vi "Iconos Indicador actual Test.vi"(8 "Test":T1 items=["Power", "Oscilloscope", "Pulse Generator", "Link FT232", "Default Reg", "W/R REG", "ADC", "Max P Min N", "Min P Max N", "Digital Offset", "Analog Offset", "Rate Scan", "Rate Scan ADD"], 9 "Icon":T2, 10 "Vasic Actual":i32, 11 "Result Test IN":T3 {"Voltage ASIC" format="%1_3g"}) -> (3 "Result Test OUT":T3 {"Voltage ASIC" format="%1_3g"})   [LabVIEW 2019]
uses:
  test check 2.ctl
  Iconos indicador actual test.ctl
  Test check.ctl
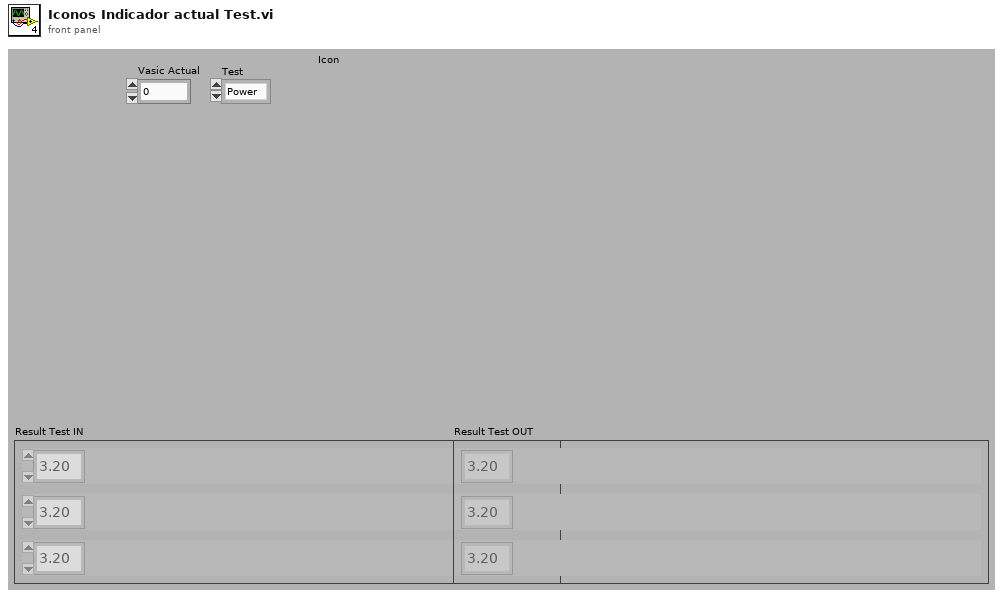
[diagram p1: front panel]
types:
  T1 = typedef "Test check.ctl" = u16
  T2 = typedef "Iconos indicador actual test.ctl" = u16
  T3 = typedef "test check 2.ctl" = cluster{"Voltage ASIC":dbl, "Power Supply":T2, "Board Test. Link Osci":T2, "Board Test. Link Gen":T2, "Board Test. Link FT232":T2, "Asic Default Registers":T2, "Asic W/R Registers":T2, "Board Test. ADC":T2, "Asic Max P Min N":T2, "Asic Min P Max N":T2, "Asic Rate Scan":T2, "Asic Rate Scan Adders":T2, "Asic Analog Offset":T2, "Asic Digital Offset":T2}[]
  T4 = cluster{"Voltage ASIC":dbl, "Power Supply":T2, "Board Test. Link Osci":T2, "Board Test. Link Gen":T2, "Board Test. Link FT232":T2, "Asic Default Registers":T2, "Asic W/R Registers":T2, "Board Test. ADC":T2, "Asic Max P Min N":T2, "Asic Min P Max N":T2, "Asic Rate Scan":T2, "Asic Rate Scan Adders":T2, "Asic Analog Offset":T2, "Asic Digital Offset":T2}
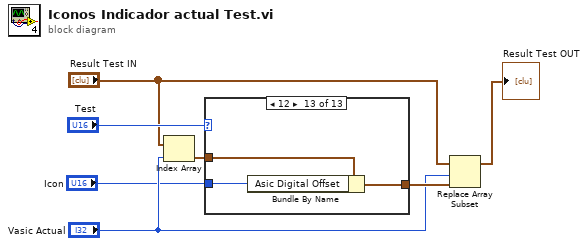
[diagram p0: block diagram]
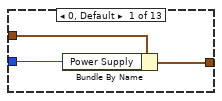
[diagram p2: hidden frame]
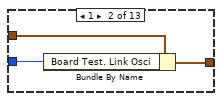
[diagram p3: hidden frame]
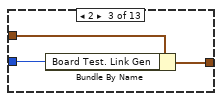
[diagram p4: hidden frame]
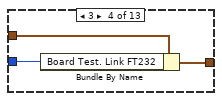
[diagram p5: hidden frame]
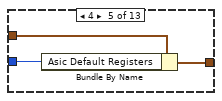
[diagram p6: hidden frame]
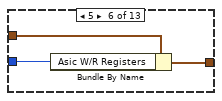
[diagram p7: hidden frame]
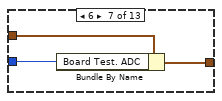
[diagram p8: hidden frame]
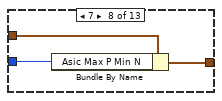
[diagram p9: hidden frame]
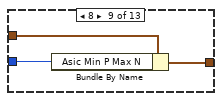
[diagram p10: hidden frame]
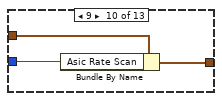
[diagram p11: hidden frame]
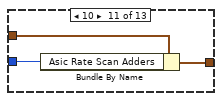
[diagram p12: hidden frame]
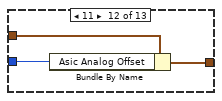
[diagram p13: hidden frame]
diagram:
  n1 = Index Array(array="Result Test IN", index="Vasic Actual") -> (element=w1:T4)
  n2 = case shown="12" "Test" {
    tunnel: w1 -> [w10 w13 w16 w19 w22 w25 w28 w31 w34 w37 w40 w43 w46]
    tunnel: "Icon" -> [w9 w12 w15 w18 w21 w24 w27 w30 w33 w36 w39 w42 w45]
    tunnel: [w8 w11 w14 w17 w20 w23 w26 w29 w32 w35 w38 w41 w44] -> w7
    frame 0, Default {
      n3 = Bundle By Name(cluster=w10, "Power Supply"=w9) -> (w8:T4)
    }
    frame 1 {
      n4 = Bundle By Name(cluster=w13, "Board Test. Link Osci"=w12) -> (w11:T4)
    }
    frame 2 {
      n5 = Bundle By Name(cluster=w16, "Board Test. Link Gen"=w15) -> (w14:T4)
    }
    frame 3 {
      n6 = Bundle By Name(cluster=w19, "Board Test. Link FT232"=w18) -> (w17:T4)
    }
    frame 4 {
      n7 = Bundle By Name(cluster=w22, "Asic Default Registers"=w21) -> (w20:T4)
    }
    frame 5 {
      n8 = Bundle By Name(cluster=w25, "Asic W/R Registers"=w24) -> (w23:T4)
    }
    frame 6 {
      n9 = Bundle By Name(cluster=w28, "Board Test. ADC"=w27) -> (w26:T4)
    }
    frame 7 {
      n10 = Bundle By Name(cluster=w31, "Asic Max P Min N"=w30) -> (w29:T4)
    }
    frame 8 {
      n11 = Bundle By Name(cluster=w34, "Asic Min P Max N"=w33) -> (w32:T4)
    }
    frame 9 {
      n12 = Bundle By Name(cluster=w37, "Asic Rate Scan"=w36) -> (w35:T4)
    }
    frame 10 {
      n13 = Bundle By Name(cluster=w40, "Asic Rate Scan Adders"=w39) -> (w38:T4)
    }
    frame 11 {
      n14 = Bundle By Name(cluster=w43, "Asic Analog Offset"=w42) -> (w41:T4)
    }
    frame 12 {
      n15 = Bundle By Name(cluster=w46, "Asic Digital Offset"=w45) -> (w44:T4)
    }
  }
  n16 = Replace Array Subset(array="Result Test IN", new element=w7, index="Vasic Actual") -> (→"Result Test OUT":T3)
